vi "Customize VI Window.vi"() -> ()   [LabVIEW 2010]
doc: "이 VI는 메뉴 모음 보이기?, 제목 표시줄 보이기?, VI를 투명하게 만들기?, VI를 가운데로와 같은 서버 메소드와 프로퍼티를 보여줍니다."
panel:
  in  "VI를 가운데로":bool
  in  "정지":bool
  in  "VI를 투명하게 만들기?":bool
  in  "제목 표시줄 보이기?":bool
  in  "메뉴 모음 보이기?":bool
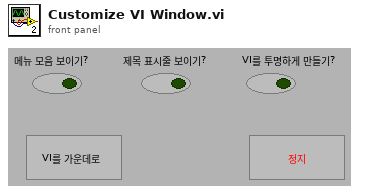
[diagram p1: front panel]
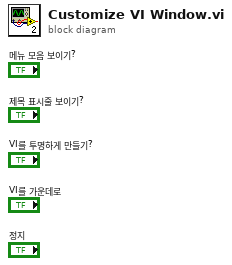
[diagram p0: block diagram]
diagram:
